vi "Wejscia.vi"(3 "Akcja":T3, 5 "Wejœcie":T1) -> (2 "Wyjœcie":T1)   [LabVIEW 2014]
uses:
  glownaMaszynaStanowVIs/AkcjaGFV.ctl
  WejsciaVIs/WejsciaParametry.ctl
  glownaMaszynaStanowVIs/wczytajListePunktowVIs/RodzajPomiarow.ctl
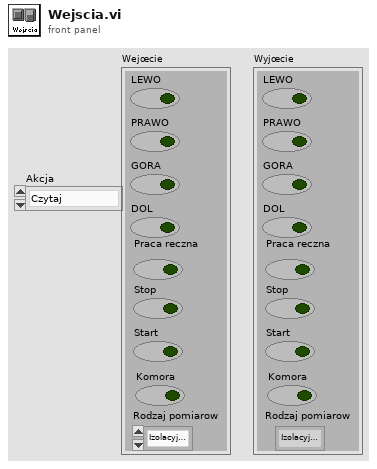
[diagram p1: front panel]
types:
  T1 = typedef "WejsciaParametry.ctl" = cluster{"LEWO":bool, "PRAWO":bool, "GORA":bool, "DOL":bool, "Stop":bool, "Start":bool, "Praca reczna":bool, "Komora":bool, "Rodzaj pomiarow":T2}
  T2 = typedef "RodzajPomiarow.ctl" = enum16{"Izolacyjnoœæ Akustyczna"}
  T3 = typedef "AkcjaGFV.ctl" = enum16{"Czytaj", "Zapisz", "Reset"}
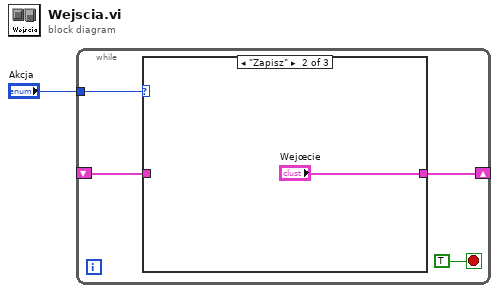
[diagram p0: block diagram]
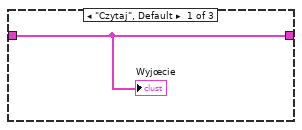
[diagram p2: hidden frame]
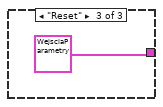
[diagram p3: hidden frame]
diagram:
  n1 = while {
    shift-right: [w3] -> _
    shift-left: _ -> [w2]
    tunnel: "Akcja" -> [w4]
    stop <- TRUE stop-if-true
    n2 = case shown="\"Zapisz\"" w4 {
      tunnel: [w6 "Wejœcie" T1 {"LEWO"=FALSE, "PRAWO"=FALSE, "GORA"=FALSE, "DOL"=FALSE, "Stop"=FALSE, "Start"=FALSE, "Praca reczna"=FALSE, "Komora"=FALSE, "Rodzaj pomiarow"=enum."Izolacyjnoœæ Akustyczna"} ("Wejœcie")] -> w3
      tunnel: w2 -> [w6 _ _]
      frame "Czytaj", Default {
        "Wyjœcie" <- w6
      }
      frame "Zapisz" {
      }
      frame "Reset" {
      }
    }
  }
